vi "Valid Image Path Check.vi"(10 "Path In":path=path "") -> (0 "error out":errorcluster)   [LabVIEW 2020]
uses:
  <userlib>/_OpenG.lib/file/file.llb/Valid Path - Traditional__ogtk.vi
  <vilib>/addons/_JKI Toolkits/Caraya/classes/Assert/Assert True.vi
  <vilib>/addons/_JKI Toolkits/Caraya/classes/Test/Test.lvclass
  <vilib>/addons/_JKI Toolkits/Caraya/classes/Assert/Assert.lvclass
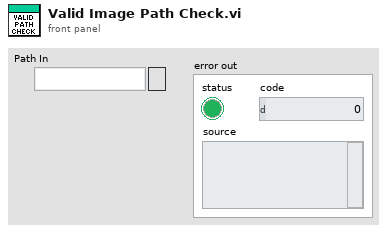
[diagram p1: front panel]
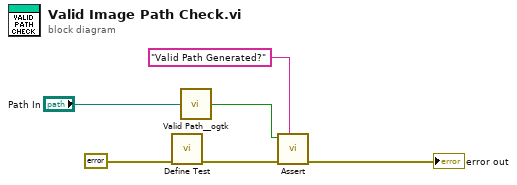
[diagram p0: block diagram]
diagram:
  n1 = call <vilib>:"Define Test.vi"("error in (no error)"=errorcluster {"status"=FALSE, "code"=0, "source"=""}) -> ("error out"=w5:errorcluster)  [unwired: 10 in]
  n2 = call-poly <userlib>:"Valid Path__ogtk.vi"("path"="Path In") -> ("valid"=w3:bool)
  n3 = call-poly <vilib>:"Assert.vi"("Label"="Valid Path Generated?" ("Label (VI Title)"), "error in (no error)"=w5, "True?"=w3) -> ("error out"=→"error out":errorcluster)  [unwired: 8 in]
